vi "Write Update Rate.vi"(8 "error in (no error)":errorcluster, 10 "Update Rate":dbl, 11 "DAQmx-Bus in":refnum<class "DAQmx-Bus.lvclass">) -> (0 "error out":errorcluster, 3 "DAQmx-Bus out":refnum<class "DAQmx-Bus.lvclass">)   [LabVIEW 2021, in "DAQmx-Bus.lvclass"]
uses:
  DAQmx-Bus.lvclass
  DAQmx-Bus.lvclass/DAQmx-Bus.ctl
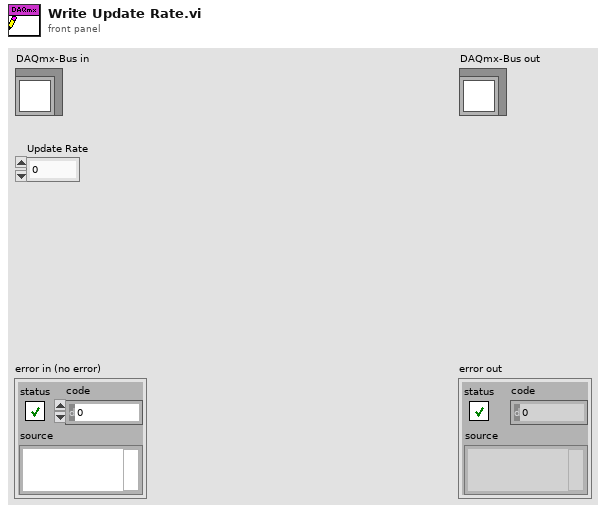
[diagram p1: front panel]
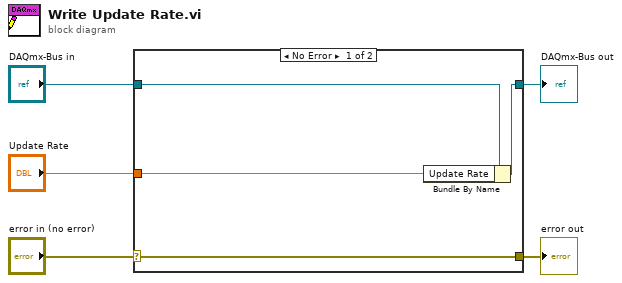
[diagram p0: block diagram]
diagram:
  n1 = case shown="No Error" "error in (no error)" {
    selector: "error in (no error)" -> [w9 w10]
    tunnel: [w9 w10] -> w4
    tunnel: [w7 w11] -> w2
    tunnel: "DAQmx-Bus in" -> [w8 w11]
    tunnel: "Update Rate" -> [w6 _]
    frame No Error {
      n2 = Bundle By Name(cluster=w8, "Update Rate"=w6) -> (w7:refnum<class "DAQmx-Bus.lvclass">)
    }
    frame Error {
    }
  }
  "error out" <- w4
  "DAQmx-Bus out" <- w2
